vi "ExPluginRead.vi"(7 "LabVIEW Web Service Request":refnum<class "Web Request.lvclass">) -> ()   [LabVIEW 2018]
uses:
  <vilib>/wsapi/Web Request.lvclass
  Lib/STM/ExPlugin/MOKO_ExPlugin_ExPlugin_STM.ctl
  Lib/STM/ExPlugin/MOKO_ExPlugin_ExPlugin_ITEM.ctl
panel:
  out "Error Out":errorcluster
  out "value":string
  # "Use the Web Service Request input terminal to call the VIs on the Web Services palette. Do not remove it from the connector pane unless you don't need access to the palette."
  # "Each additional control wired to the connector pane will be available as an input in the URL. To include an indicator in terminal-mode output (the default setting), it must also be wired to the connector pane."
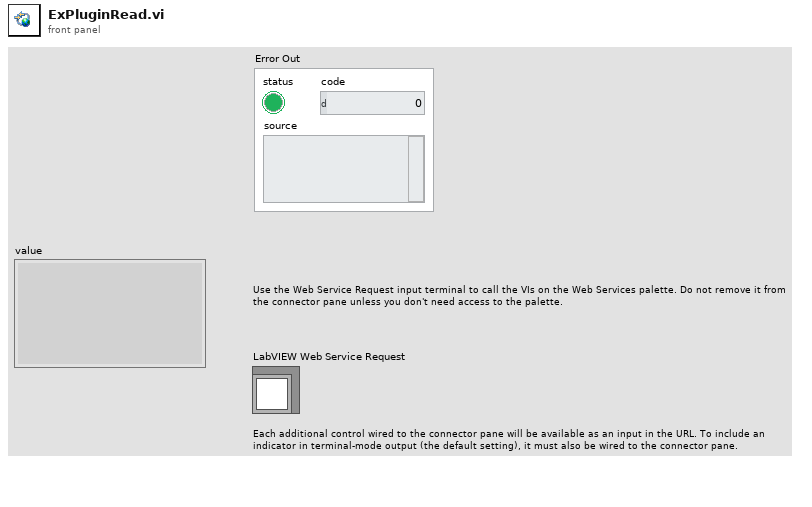
[diagram p1: front panel]
types:
  T1 = typedef "MOKO_ExPlugin_ExPlugin_ITEM.ctl" = enum16{"idle", "ExPlugin read", "ExPlugin write"}
  T2 = typedef "MOKO_ExPlugin_ExPlugin_STM.ctl" = cluster{"main stm":T1, "data":string}
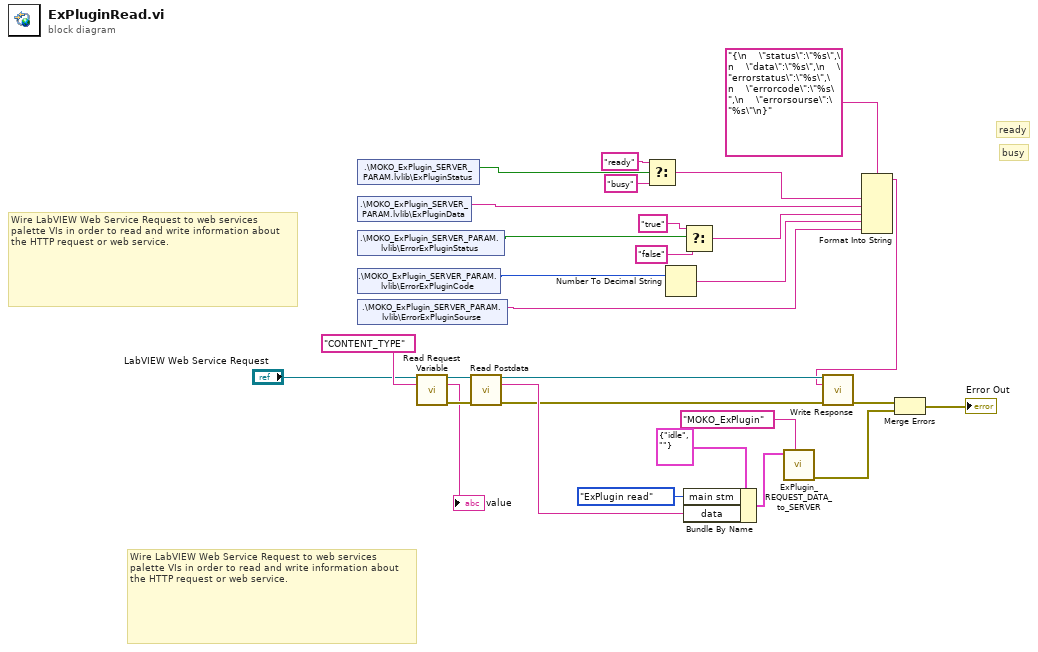
[diagram p0: block diagram]
diagram:
  # "busy"
  # "ready"
  # "Wire LabVIEW Web Service Request to web services palette VIs in order to read and write information about the HTTP request or web service."
  # "Wire LabVIEW Web Service Request to web services palette VIs in order to read and write information about the HTTP request or web service."
  n1 = shared-variable ".\\MOKO_ExPlugin_SERVER_PARAM.lvlib\\ExPluginStatus"() -> (w5:bool)  [unwired: 1 in, 1 out]
  n2 = shared-variable ".\\MOKO_ExPlugin_SERVER_PARAM.lvlib\\ExPluginData"() -> (w4:string)  [unwired: 1 in, 1 out]
  n3 = shared-variable ".\\MOKO_ExPlugin_SERVER_PARAM.lvlib\\ErrorExPluginStatus"() -> (w3:bool)  [unwired: 1 in, 1 out]
  n4 = shared-variable ".\\MOKO_ExPlugin_SERVER_PARAM.lvlib\\ErrorExPluginCode"() -> (w2:i32)  [unwired: 1 in, 1 out]
  n5 = shared-variable ".\\MOKO_ExPlugin_SERVER_PARAM.lvlib\\ErrorExPluginSourse"() -> (w1:string)  [unwired: 1 in, 1 out]
  n6 = call <vilib>:"Read Request Variable.vi"("LabVIEW Web Service Request"="LabVIEW Web Service Request", "variable name"="CONTENT_TYPE") -> ("LabVIEW Web Service Request out"=w28:refnum<class "Web Request.lvclass">, "value"=→"value":string, "error out"=w27:errorcluster)  [unwired: 11 in]
  n7 = call <vilib>:"Read Postdata.vi"("LabVIEW Web Service Request"=w28, "error in (no error)"=w27) -> ("LabVIEW Web Service Request out"=w23:refnum<class "Web Request.lvclass">, "postdata"=w26:string, "error out"=w22:errorcluster)  [unwired: 11 in]
  n8 = Select(t="ready", s=w5, f="busy") -> (s? t:f=w14:string)
  n9 = Number To Decimal String(number=w2) -> (decimal integer string=w10:string)  [unwired: 1 in]
  n10 = Select(t="true", s=w3, f="false") -> (s? t:f=w11:string)
  n11 = Bundle By Name(cluster=T2 {"main stm"=enum."idle", "data"=""} ("MOKO_NMEA"), "main stm"=MOKO_ExPlugin_ExPlugin_ITEM."ExPlugin read", "data"=w26) -> (w21:T2)
  n12 = call "ExPlugin_REQUEST_DATA_to_SERVER.vi"("Control Name"="MOKO_ExPlugin", "MOKO_ExPlugin_STM"=w21) -> ("Error Out"=w24:errorcluster)  [unwired: 9 in]
  n13 = Format Into String(format string="{\n    \"status\":\"%s\",\n    \"data\":\"%s\",\n    \"errorstatus\":\"%s\",\n    \"errorcode\":\"%s\",\n    \"errorsourse\":\"%s\"\n}", w14, w4, w11, w10, w1) -> (resulting string=w17:string)  [unwired: 2 in, 1 out]
  n14 = call <vilib>:"Write Response.vi"("LabVIEW Web Service Request"=w23, "response string"=w17, "error in (no error)"=w22) -> ("error out"=w20:errorcluster)  [unwired: 11 in, 1 out]
  n15 = Merge Errors(w20, w24) -> (→"Error Out":errorcluster)
